vi "Get UI Details.vi"() -> ()   [LabVIEW 2023, in "LabVIEW Bodeplot Summit.lvlib"]
uses:
  LabVIEW Bodeplot Summit.lvlib
  <vilib>/MeasurementLink/MeasurementLink Measurement Server/Helpers/TypeDefs/UI Information.ctl
  <vilib>/MeasurementLink/MeasurementLink Measurement Server/MeasurementLink Measurement Server.lvlib
panel:
  out "error out":errorcluster
  in  "error in (no error)":errorcluster
  out "UI Details":T1[](array[typedef])
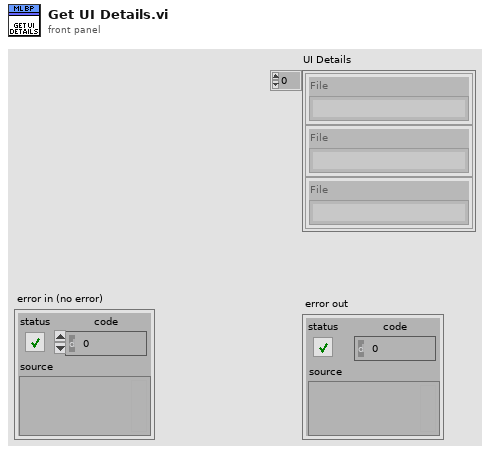
[diagram p1: front panel]
types:
  T1 = typedef "MeasurementLink Measurement Server.lvlib/UI Information.ctl" = cluster{"File":string}
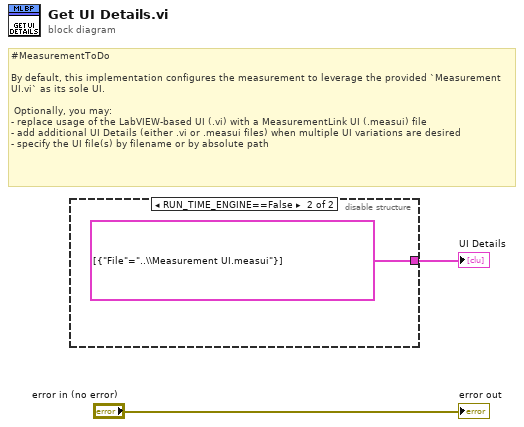
[diagram p0: block diagram]
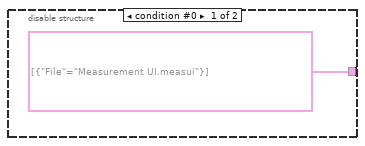
[diagram p2: hidden frame]
diagram:
  # "#MeasurementToDo\n\nBy default, this implementation configures the measurement to leverage the provided `Measurement UI.vi` as its sole UI.\n\n Optionally, you may:\n- replace usage of the LabVIEW-based UI (.vi) with a MeasurementLink UI (.measui) file\n- add additional UI Details (either .vi or .measui files) when multiple UI variations are desired\n- specify the UI file(s) by filename or by absolute path"
  n1 = disable-structure shown="RUN_TIME_ENGINE==False" {
    disable-tunnel: [T1[] [{"File"="Measurement UI.measui"}] ("appended array") T1[] [{"File"="..\\Measurement UI.measui"}] ("appended array")] -> w2
    frame condition #0 {
    }
    frame condition #1 (active) {
    }
  }
  "UI Details" <- w2
  "error out" <- "error in (no error)"
